vi "更新程序.vi"() -> ()   [LabVIEW 2016, in "自动更新.lvlib"]
uses:
  <vilib>/FTP/NI_FTP.lvlib
panel:
  out "软件版本 2":string caption="目标软件版本"
  out "软件版本":string caption="当前软件版本"
  out "下载的文件名":string
  out "目标文件夹名":string
  out "端口号":i32
  out "IP地址":string
  out "步骤":string
  out "当前步骤":string
  in  "目标路径（使用对话框）":path
  out "下载保存目录":path
  out "更新进度":u8(slide) scale=0.0..100.0
  # "1.先下载更新-------2.关闭主应用-------3.替换应用--------4.打开主应用-----------5.关闭本程序"
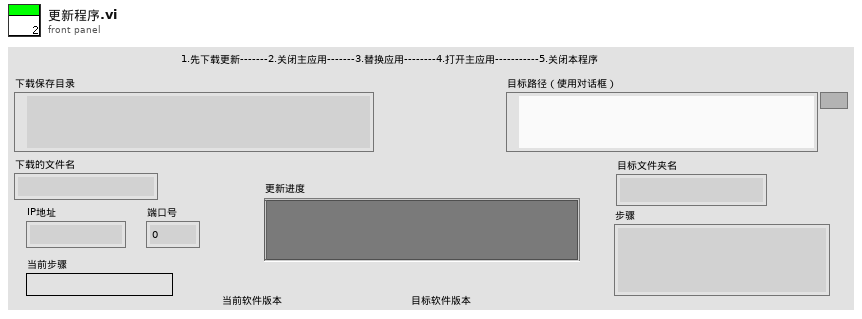
[diagram p1: front panel]
types:
  T1 = enum16{"open", "replace", "create", "open or create", "replace or create", "replace or create with confirmation"}
  T2 = cluster{"网络灯":bool, "接收中":bool, "已接收百分比":u8, "接收成功次数":dbl, "当前步骤":enum16{"init", "receivehead", "receivecontent", "receivesuccess", "over"}, "文件名":string, "error out":errorcluster}
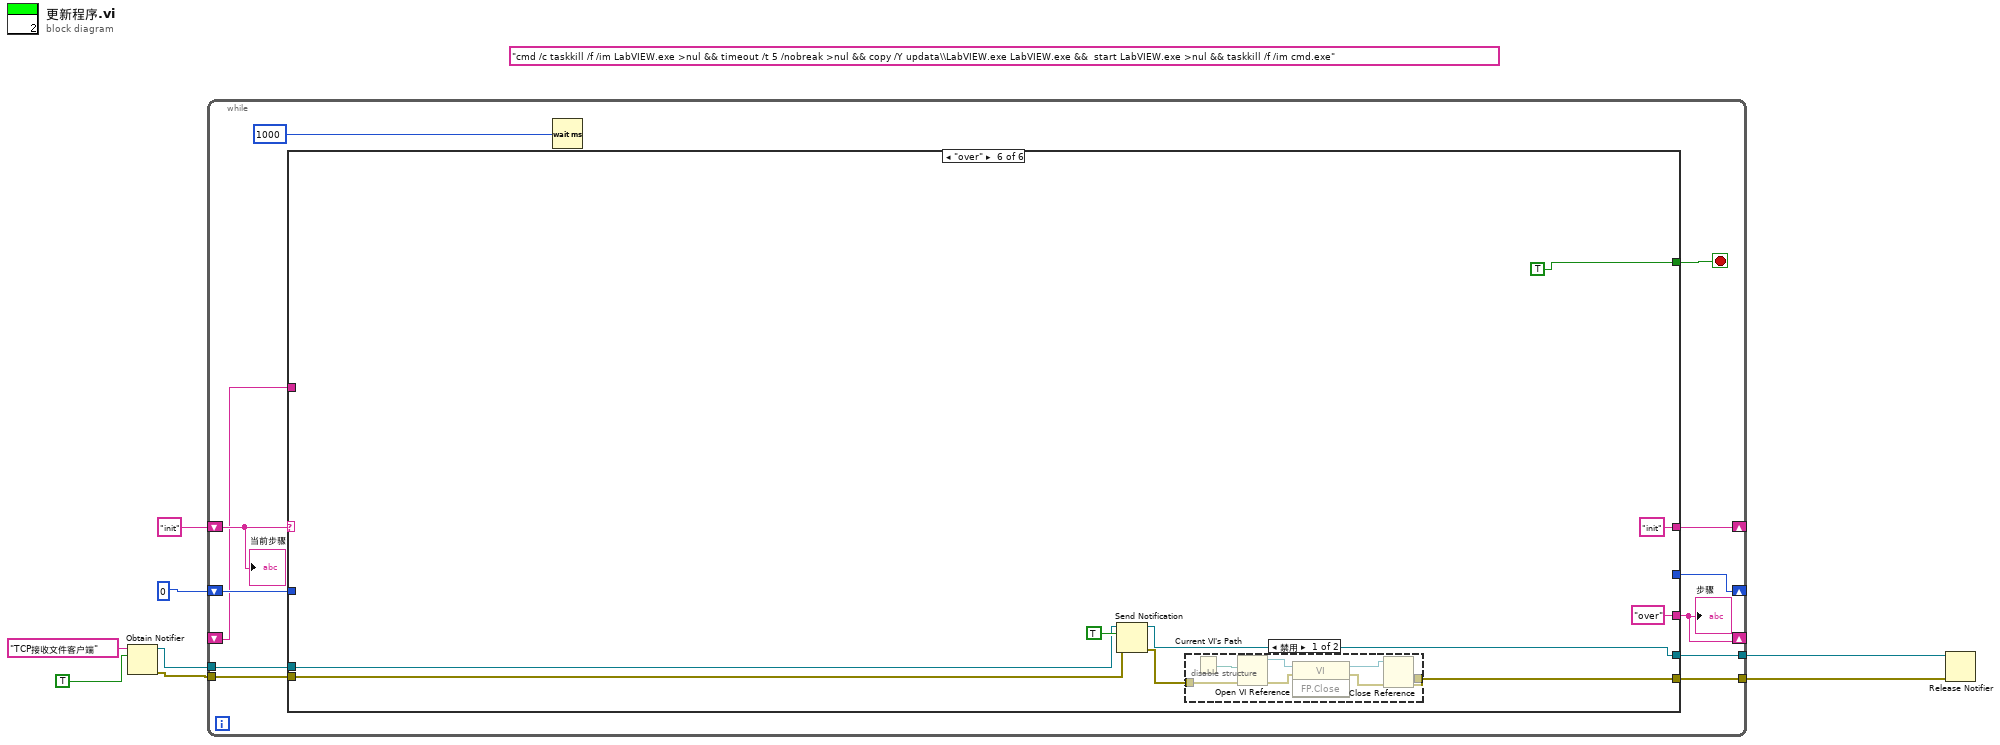
[diagram p0: block diagram]
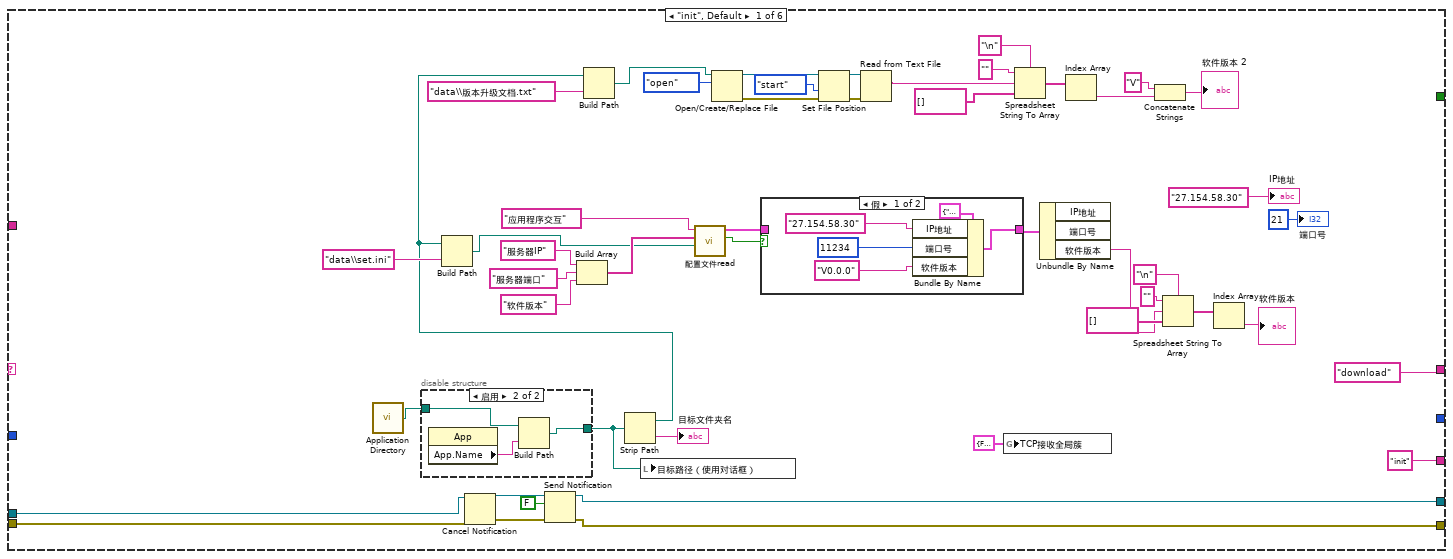
[diagram p2: hidden frame]
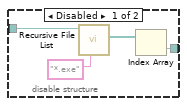
[diagram p3: hidden frame]
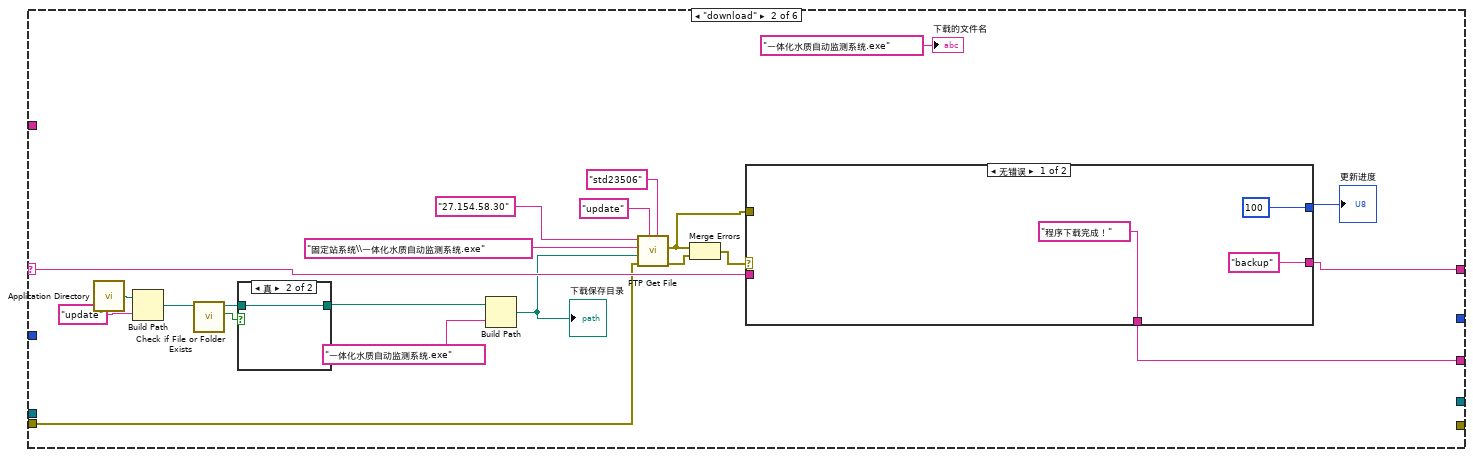
[diagram p5: hidden frame]
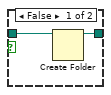
[diagram p6: hidden frame]
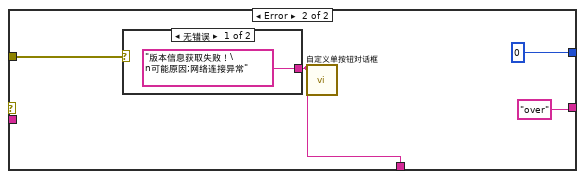
[diagram p7: hidden frame]
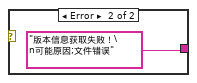
[diagram p8: hidden frame]
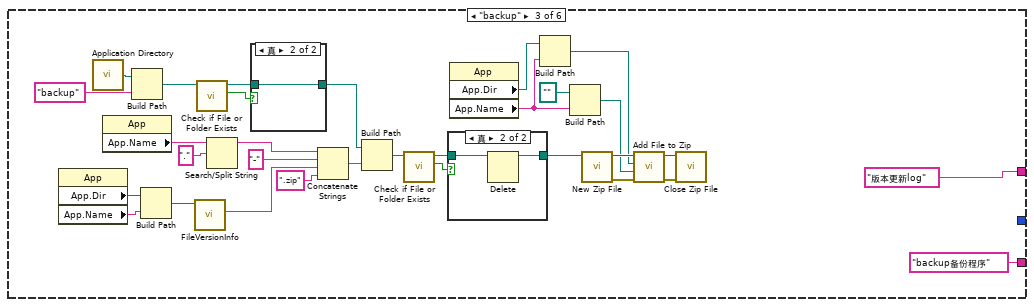
[diagram p9: hidden frame]
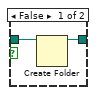
[diagram p11: hidden frame]
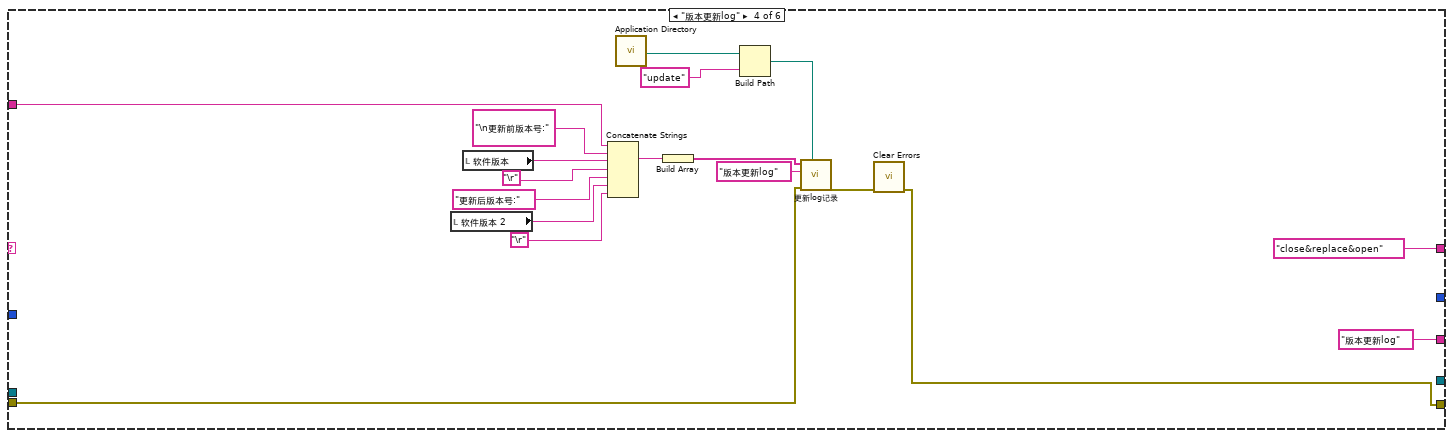
[diagram p12: hidden frame]
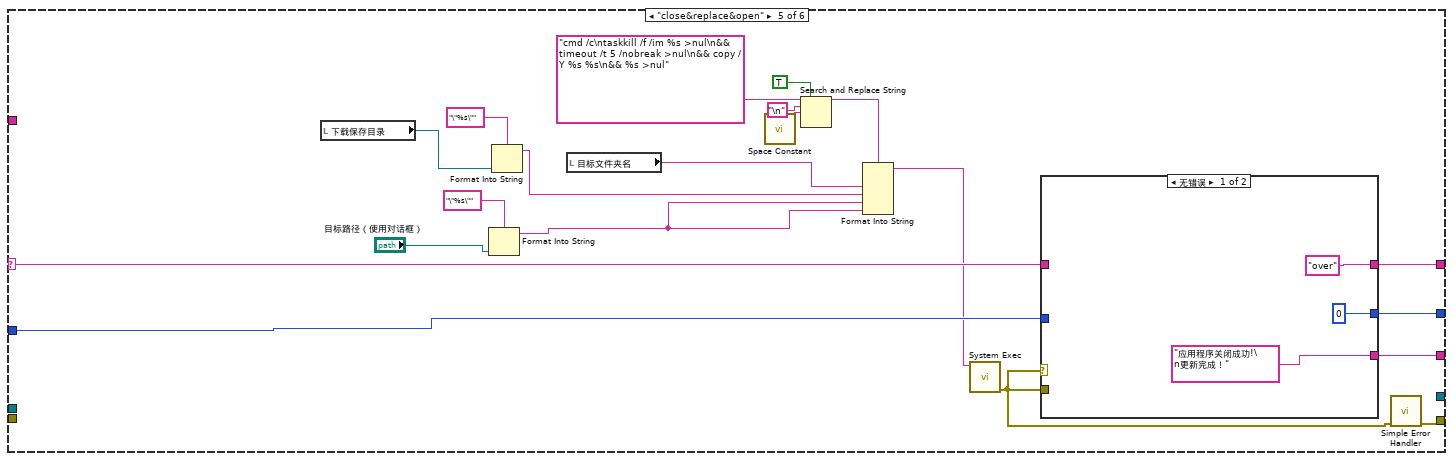
[diagram p13: hidden frame]
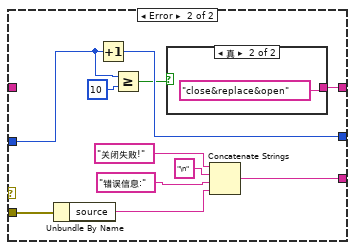
[diagram p14: hidden frame]
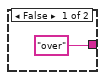
[diagram p15: hidden frame]
diagram:
  (unwired) "cmd /c taskkill /f /im LabVIEW.exe >nul && timeout /t 5 /nobreak >nul && copy /Y updata\\LabVIEW.exe LabVIEW.exe &&  start LabVIEW.exe >nul && taskkill /f /im cmd.exe" ("结果字符串")
  n1 = Obtain Notifier(name (unnamed)="TCP接收文件客户端" ("名称（未命名）"), notification data type=TRUE) -> (notifier out=w6:refnum<notifier>, error out=w5:errorcluster)  [unwired: 2 in, 1 out]
  n2 = while {
    shift-right: [w19] -> _
    shift-left: "init" -> [w20]
    tunnel: w6 -> [w16]
    tunnel: w5 -> [w15]
    tunnel: [w14] -> w4
    tunnel: [w13] -> w3
    shift-right: [w11] -> _
    shift-left: u8 0 -> [w12]
    shift-right: [w10] -> _
    shift-left: _ -> [w9]
    stop <- w18 stop-if-true
    n3 = case shown="\"over\"" w20 {
      selector: w20 -> [_ w92 _ _ w189 _]
      tunnel: ["download" w93 "版本更新log" "close&replace&open" w188 "init"] -> w19
      tunnel: [_ _ _ _ _ TRUE] -> w18
      tunnel: ["init" ("步骤") w90 "backup备份程序" ("步骤") "版本更新log" ("步骤") w187 "over" ("步骤")] -> w10
      tunnel: w16 -> [w67 _ _ _ _ w212]
      tunnel: w15 -> [w66 w91 _ w162 _ w211]
      tunnel: [w62 _ _ _ _ w210] -> w14
      tunnel: [w61 _ _ w152 w171 w209] -> w13
      tunnel: w12 -> [_ _ _ _ w186 _]
      tunnel: [_ _ _ _ w185 _] -> w11
      tunnel: w9 -> [_ _ _ w157 _ _]
      frame "init", Default {
        n4 = call <vilib>:"Application Directory.vi"() -> ("Application Directory"=w22:path)
        n5 = disable-structure shown="启用" {
          disable-tunnel: [w72 w73] -> w59
          disable-tunnel: w22 -> [w69 w75]
          frame Disabled {
            n6 = call <vilib>:"Recursive File List.vi"("pattern"="*.exe", "Folder Path"=w69) -> ("All Files in Dir"=w71:path[])  [unwired: 5 in, 4 out]
            n7 = Index Array(array=w71) -> (element=w72:path)  [unwired: 1 in]
          }
          frame Enabled {
            n8 = property class="App"() -> ("App.Name"=w74:string)  [unwired: 2 in, 2 out]
            n9 = Build Path(base path=w75, name or relative path=w74) -> (appended path=w73:path)
          }
        }
        n10 = Cancel Notification(0:w67, 3:w66) -> (8:w65:refnum<notifier>, 11:w63:errorcluster)  [unwired: 1 out]
        n11 = Send Notification(notification=FALSE ("通知"), notifier=w65, error in (no error)=w63) -> (notifier out=w62:refnum<notifier>, error out=w61:errorcluster)
        n12 = Build Array("服务器IP" ("section"), "服务器端口" ("section"), "软件版本" ("key")) -> (w31:string[])
        n13 = Strip Path(path=w59) -> (stripped path=w35:path, name=→"目标文件夹名":string)
        n14 = Build Path(base path=w35, name or relative path="data\\set.ini" ("名称或相对路径")) -> (appended path=w27:path)
        n15 = Build Path(base path=w35, name or relative path="data\\版本升级文档.txt" ("名称或相对路径")) -> (appended path=w43:path)
        n16 = local write "目标路径（使用对话框）"(w59) -> ()
        n17 = call "配置文件read.vi"("configuration file path"=w27, "键数组"=w31, "段"="应用程序交互" ("section")) -> ("section exists?"=w33:bool, "updateconfiguration"=w34:cluster{"IP地址":string, "端口号":i32, "软件版本":string})  [unwired: 6 in, 1 out]
        n18 = Open/Create/Replace File(file path (use dialog)=w43, operation (0:open)=T1."open" ("操作(0:open)")) -> (refnum out=w38:refnum<file>, error out=w39:errorcluster)  [unwired: 4 in, 1 out]
        n19 = case shown="假" w33 {
          tunnel: w34 -> [_ w81]
          tunnel: [w76 w81] -> w26
          frame False {
            n20 = Bundle By Name(cluster=cluster{"IP地址":string, "端口号":i32, "软件版本":string} {"IP地址"="", "端口号"=0, "软件版本"=""} ("updateconfiguration"), "IP地址"="27.154.58.30" ("key"), "端口号"=11234 ("value"), "软件版本"="V0.0.0" ("key")) -> (w76:cluster{"IP地址":string, "端口号":i32, "软件版本":string})
          }
          frame True {
          }
        }
        n21 = Set File Position(refnum=w38, from (0:start)=enum16{"start", "end", "current"}."start" ("自（0:起始）"), error in=w39) -> (refnum out=w42:refnum<file>, error out=w40:errorcluster)  [unwired: 1 in]
        n22 = Read from Text File(file (use dialog)=w42, error in=w40) -> (text=w50:string)  [unwired: 2 in, 3 out]
        n23 = global write "全局变量1.vi" "TCP接收全局簇"(T2 {"网络灯"=FALSE, "接收中"=FALSE, "已接收百分比"=0, "接收成功次数"=0.0, "当前步骤"=enum."init", "文件名"="", "error out"={"status"=FALSE, "code"=0, "source"=""}} ("TCP接收全局簇")) -> ()
        n24 = Spreadsheet String To Array(delimiter (Tab)="\n" ("分隔符(Tab)"), format string="" ("格式字符串"), spreadsheet string=w50, array type (2D Dbl)=string[] []) -> (array=w47:string[])
        n25 = Unbundle By Name(w26) -> ("软件版本"=w25:string)  [unwired: 2 out]
        n26 = Index Array(array=w47) -> (element=w48:string)  [unwired: 1 in]
        n27 = Concatenate Strings("V" ("字符串"), w48) -> (→"软件版本 2":string)
        n28 = Spreadsheet String To Array(delimiter (Tab)="\n" ("分隔符(Tab)"), format string="" ("格式字符串"), spreadsheet string=w25, array type (2D Dbl)=string[] []) -> (array=w53:string[])
        n29 = Index Array(array=w53) -> (element=→"软件版本":string)  [unwired: 1 in]
        "IP地址" <- "27.154.58.30" ("key")
        "端口号" <- 21 ("端口号")
      }
      frame "download" {
        n30 = call <vilib>:"Application Directory.vi"() -> ("Application Directory"=w84:path)
        n31 = Build Path(base path=w84, name or relative path="update" ("名称或相对路径")) -> (appended path=w85:path)
        n32 = call <vilib>:"Check if File or Folder Exists.vi"("path"=w85) -> ("file or folder exists?"=w86:bool, "dup path"=w87:path)  [unwired: 8 in, 1 out]
        n33 = case shown="真" w86 {
          tunnel: w87 -> [w104 w105]
          tunnel: [w103 w105] -> w82
          frame False {
            n34 = Create Folder(path (use dialog)=w104) -> (created path=w103:path)  [unwired: 2 in, 2 out]
          }
          frame True {
          }
        }
        n35 = Build Path(base path=w82, name or relative path="一体化水质自动监测系统.exe" ("名称或相对路径")) -> (appended path=w88:path)
        "下载保存目录" <- w88
        n36 = call <vilib>:"FTP Get File.vi"("password"="std23506", "user"="update", "error in (no error)"=w91, "local path"=w88, "remote path"="固定站系统\\一体化水质自动监测系统.exe", "host"="27.154.58.30") -> ("error out"=w98:errorcluster, "file error"=w97:errorcluster)  [unwired: 4 in]
        n37 = Merge Errors(w97, w98) -> (w96:errorcluster)
        n38 = case shown="无错误" w96 {
          tunnel: w97 -> [_ w112]
          tunnel: [u8 100 ("y") u8 0 ("y")] -> w95
          tunnel: ["backup" "over"] -> w93
          tunnel: w92 -> [_ _]
          tunnel: ["程序下载完成！" w110] -> w90
          frame No Error {
          }
          frame Error {
            n39 = case shown="无错误" w112 {
              tunnel: ["版本信息获取失败！\n可能原因;网络连接异常" "版本信息获取失败！\n可能原因;文件错误"] -> w110
              frame No Error {
              }
              frame Error {
              }
            }
            n40 = call "自定义单按钮对话框.vi"("消息"=w110) -> ()  [unwired: 11 in]
          }
        }
        "更新进度" <- w95
        "下载的文件名" <- "一体化水质自动监测系统.exe" ("下载的文件名")
      }
      frame "backup" {
        n41 = property class="App"() -> ("App.Dir"=w137:path, "App.Name"=w143:string)  [unwired: 2 in, 2 out]
        n42 = call <vilib>:"Application Directory.vi"() -> ("Application Directory"=w144:path)
        n43 = property class="App"() -> ("App.Name"=w141:string)  [unwired: 2 in, 2 out]
        n44 = Build Path(base path=w144, name or relative path="backup" ("名称或相对路径")) -> (appended path=w124:path)
        n45 = Build Path(base path=w137, name or relative path=w143) -> (appended path=w142:path)
        n46 = call <vilib>:"FileVersionInfo.vi"("Application Path in"=w142) -> ("File Version Info"=w139:string)  [unwired: 7 in, 3 out]
        n47 = call <vilib>:"Check if File or Folder Exists.vi"("path"=w124) -> ("file or folder exists?"=w123:bool, "dup path"=w122:path)  [unwired: 8 in, 1 out]
        n48 = Search/Split String(string=w141, search string/char (-)="." ("搜索字符串/字符(-)")) -> (substring before match=w135:string)  [unwired: 1 in, 2 out]
        n49 = case shown="真" w123 {
          tunnel: w122 -> [w150 w151]
          tunnel: [w149 w151] -> w121
          frame False {
            n50 = Create Folder(path (use dialog)=w150) -> (created path=w149:path)  [unwired: 2 in, 2 out]
          }
          frame True {
          }
        }
        n51 = Concatenate Strings(w135, "-" ("字符串"), w139, ".zip" ("字符串")) -> (w134:string)
        n52 = Build Path(base path=w121, name or relative path=w134) -> (appended path=w118:path)
        n53 = call <vilib>:"Check if File or Folder Exists.vi"("path"=w118) -> ("file or folder exists?"=w119:bool, "dup path"=w120:path)  [unwired: 8 in, 1 out]
        n54 = case shown="真" w119 {
          tunnel: w120 -> [w146 w148]
          tunnel: [w146 w147] -> w117
          frame False {
          }
          frame True {
            n55 = Delete(path (use dialog)=w148) -> (deleted path=w147:path)  [unwired: 4 in, 2 out]
          }
        }
        n56 = property class="App"() -> ("App.Dir"=w133:path, "App.Name"=w126:string)  [unwired: 2 in, 2 out]
        n57 = Build Path(base path=w133, name or relative path=w126) -> (appended path=w128:path)
        n58 = Build Path(base path=path "" ("Relative Path from 1 to 2"), name or relative path=w126) -> (appended path=w125:path)
        n59 = call <vilib>:"New Zip File.vi"("target"=w117) -> ("error out"=w132:errorcluster, "zip file out"=w131:i64)  [unwired: 2 in, 3 out]
        n60 = call <vilib>:"Add File to Zip.vi"("error in (no error)"=w132, "destination path in zip"=w125, "source file path"=w128, "zip file in"=w131) -> ("error out"=w129:errorcluster, "zip file out"=w130:i64)  [unwired: 6 in]
        n61 = call <vilib>:"Close Zip File.vi"("error in (no error)"=w129, "zip file in"=w130) -> ()  [unwired: 5 in, 1 out]
      }
      frame "版本更新log" {
        n62 = local read "软件版本 2"() -> (w159:string)
        n63 = local read "软件版本"() -> (w161:string)
        n64 = Concatenate Strings(w157, "\n更新前版本号:" ("字符串"), w161, "\r", "更新后版本号:", w159, "\r") -> (w167:string)
        n65 = call <vilib>:"Application Directory.vi"() -> ("Application Directory"=w155:path)
        n66 = Build Array(w167) -> (w166:string[])
        n67 = Build Path(base path=w155, name or relative path="update" ("名称或相对路径")) -> (appended path=w154:path)
        n68 = call "更新log记录.vi"("路径"=w154, "错误输入（无错误）"=w162, "logname"="版本更新log", "数组"=w166) -> ("错误输出"=w163:errorcluster)  [unwired: 7 in]
        n69 = call <vilib>:"Clear Errors.vi"("error in (no error)"=w163) -> ("error out"=w152:errorcluster)  [unwired: 5 in, 1 out]
      }
      frame "close&replace&open" {
        n70 = local read "下载保存目录"() -> (w177:path)
        n71 = Format Into String(format string="\"%s\"" ("格式字符串"), "目标路径（使用对话框）") -> (resulting string=w173:string)  [unwired: 2 in, 1 out]
        n72 = Format Into String(format string="\"%s\"" ("格式字符串"), w177) -> (resulting string=w175:string)  [unwired: 2 in, 1 out]
        n73 = local read "目标文件夹名"() -> (w184:string)
        n74 = call <vilib>:"Space Constant.vi"() -> ("String"=w180:string)
        n75 = Search and Replace String(replace all?=TRUE ("替换全部？(F)"), input string="cmd /c\ntaskkill /f /im %s >nul\n&& timeout /t 5 /nobreak >nul\n&& copy /Y %s %s\n&& %s >nul" ("名称或相对路径"), search string="\n", replace string=w180) -> (result string=w183:string)  [unwired: 4 in, 3 out]
        n76 = Format Into String(format string=w183, w184, w175, w173, w173) -> (resulting string=w178:string)  [unwired: 2 in, 1 out]
        n77 = call <vilib>:"System Exec.vi"("command line"=w178) -> ("error out"=w170:errorcluster)  [unwired: 7 in, 3 out]
        n78 = case shown="无错误" w170 {
          tunnel: ["over" w197] -> w188
          tunnel: w170 -> [_ w203]
          tunnel: ["应用程序关闭成功!\n更新完成！" ("步骤") w198] -> w187
          tunnel: w189 -> [_ _]
          tunnel: w186 -> [_ w193]
          tunnel: [u8 0 w195] -> w185
          frame No Error {
          }
          frame Error {
            n79 = Unbundle By Name(w203) -> ("source"=w202:string)
            n80 = Increment(x=w193) -> (x+1=w195:u8)
            n81 = Greater Or Equal?(x=w193, y=u8 10) -> (x >= y?=w194:bool)
            n82 = case shown="真" w194 {
              tunnel: ["over" "close&replace&open"] -> w197
              frame False {
              }
              frame True {
              }
            }
            n83 = Concatenate Strings("关闭失败!" ("消息"), "\n" ("字符串"), "错误信息:" ("字符串"), w202) -> (w198:string)
          }
        }
        n84 = call <vilib>:"Simple Error Handler.vi"("error in (no error)"=w170) -> ("error out"=w171:errorcluster)  [unwired: 4 in, 4 out]
      }
      frame "over" {
        n85 = Send Notification(notification=TRUE, notifier=w212, error in (no error)=w211) -> (notifier out=w210:refnum<notifier>, error out=w213:errorcluster)
        n86 = disable-structure shown="禁用" {
          disable-tunnel: w213 -> [w218 _]
          disable-tunnel: [w215 _] -> w209
          frame Disabled {
            n87 = Current VI's Path() -> (path=w220:path)
            n88 = Open VI Reference(vi path=w220, error in (no error)=w218) -> (vi reference=w219:refnum<vi>, error out=w221:errorcluster)  [unwired: 4 in]
            n89 = invoke class="VI" method="FP.Close"(reference=w219, error in=w221) -> (reference out=w216:refnum<vi>, error out=w217:errorcluster)  [unwired: 1 in, 1 out]
            n90 = Close Reference(reference=w216, error in (no error)=w217) -> (error out=w215:errorcluster)
          }
          frame Enabled {
          }
        }
      }
    }
    "步骤" <- w10
    n91 = Wait (ms)(milliseconds to wait=u32 1000 ("等待时间（毫秒）")) -> ()  [unwired: 1 out]
    "当前步骤" <- w20
  }
  n92 = Release Notifier(notifier=w4, error in (no error)=w3) -> ()  [unwired: 1 in, 3 out]
